vi "IOC shared memory initialize.vi"(10 "Shared Memory Name":string="/labview_linux_sm", 11 "Shared Memory Size (bytes)":u32=4096) -> (0 "Shared memory cluster":T1, 3 "shared memory class":T2)   [LabVIEW 2020, in "linuxSharedMemory.lvlib"]
uses:
  linuxSharedMemory.lvlib
  <vilib>/NI/NI Linux RT IPC/Shared Memory/Controls/file mode.ctl
  <vilib>/NI/NI Linux RT IPC/Shared Memory/Controls/reference.ctl
  <vilib>/NI/NI Linux RT IPC/Shared Memory/Classes/Shared Memory/Shared Memory.lvclass
  controls/sm_cluster.ctl
  <vilib>/NI/NI Linux RT IPC/Shared Memory/Linux RT IPC.Shared Memory.lvlib
panel:
  in  "Shared memory cluster":T1
  in  "file mode (open)":T3=enum."create/replace"
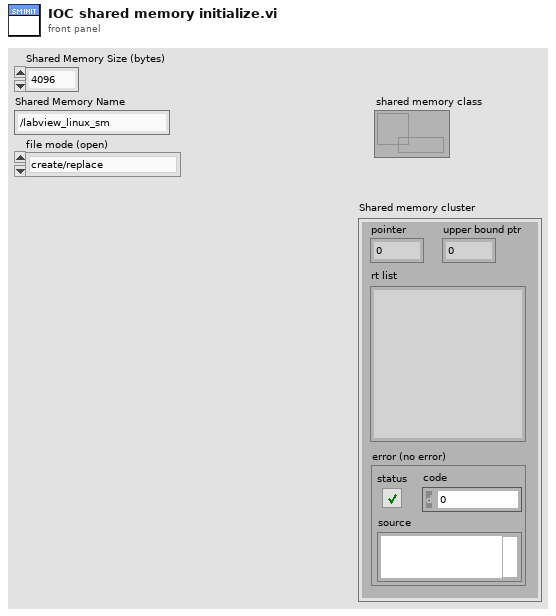
[diagram p1: front panel]
types:
  T1 = typedef "linuxSharedMemory.lvlib/sm_cluster.ctl" = cluster{"rt list":string, "error (no error)":errorcluster, "pointer":u64, "upper bound ptr":u64}
  T2 = typedef "Linux RT IPC.Shared Memory.lvlib/reference.ctl" = refnum<data-value>
  T3 = typedef "Linux RT IPC.Shared Memory.lvlib/file mode.ctl" = enum16{"open", "create/replace"}
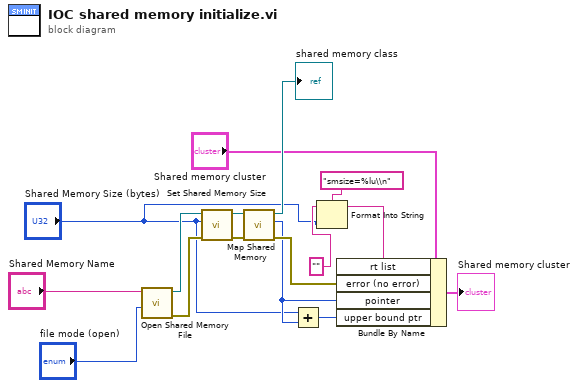
[diagram p0: block diagram]
diagram:
  n1 = call <vilib>:"Open Shared Memory File.vi"("file mode (open)"="file mode (open)", "shared memory name"="Shared Memory Name") -> ("error out"=w13:errorcluster, "shared memory out"=w14:T2)  [unwired: 8 in]
  n2 = call <vilib>:"Set Shared Memory Size.vi"("error in (no error)"=w13, "size (bytes)"="Shared Memory Size (bytes)", "shared memory in"=w14) -> ("error out"=w15:errorcluster, "shared memory out"=w16:T2)  [unwired: 7 in]
  n3 = call <vilib>:"Map Shared Memory.vi"("error in (no error)"=w15, "shared memory in"=w16) -> ("error out"=w6:errorcluster, "pointer to shared memory"=w5:u64, "shared memory out"=→"shared memory class":T2)  [unwired: 7 in]
  n4 = Add(x="Shared Memory Size (bytes)", y=w5) -> (x+y=w7:u64)
  n5 = Format Into String(format string="smsize=%lu\\n", initial string="", "Shared Memory Size (bytes)") -> (resulting string=w3:string)  [unwired: 1 in, 1 out]
  n6 = Bundle By Name(cluster="Shared memory cluster", "rt list"=w3, "error (no error)"=w6, "pointer"=w5, "upper bound ptr"=w7) -> (→"Shared memory cluster":T1)
